vi "TCP IP Parse BipolarPower.vi"(11 "JSON in":string) -> (2 "Bipolar Power Level":string, 3 "JSON out":string)   [LabVIEW 2015]
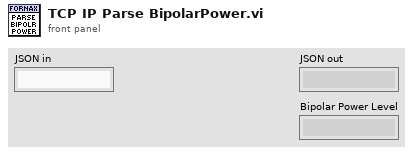
[diagram p1: front panel]
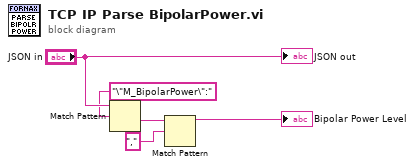
[diagram p0: block diagram]
diagram:
  n1 = Match Pattern(string="JSON in", regular expression="\"M_BipolarPower\":") -> (after substring=w2:string)  [unwired: 1 in, 3 out]
  n2 = Match Pattern(string=w2, regular expression=",") -> (before substring=→"Bipolar Power Level":string)  [unwired: 1 in, 3 out]
  "JSON out" <- "JSON in"
